vi "SHA-1.vi"(1 "Data":u8[](array[numeric])) -> (0 "message-digest":u8[](array[numeric]))   [LabVIEW 2016, in "websocket upgrade handler.lvclass"]
uses:
  websocket upgrade handler.lvclass
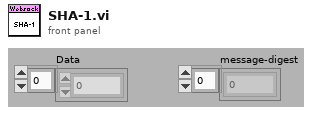
[diagram p1: front panel]
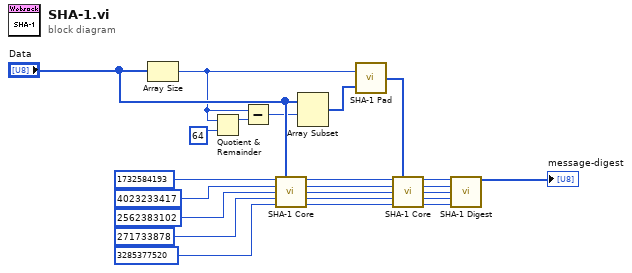
[diagram p0: block diagram]
diagram:
  n1 = Array Size(array="Data") -> (size(s)=w1:i32)
  n2 = Quotient & Remainder(x=w1, y=64) -> (x-y*floor(x/y)=w12:i32)  [unwired: 1 out]
  n3 = Subtract(x=w1, y=w12) -> (x-y=w18:i32)
  n4 = call "SHA-1 Core.vi"("s1"=u32 1732584193, "Input Bytes"="Data", "s2"=u32 4023233417, "s3"=u32 2562383102, "s4"=u32 271733878, "s5"=u32 3285377520 ("s4")) -> ("s1 out"=w13:u32, "s2 out"=w14:u32, "s3 out"=w15:u32, "s4 out"=w16:u32, "s5 out"=w17:u32)  [unwired: 5 in]
  n5 = Array Subset(array="Data", index=w18) -> (w19:u8[])  [unwired: 1 in]
  n6 = call "SHA-1 Pad.vi"("Last Part"=w19, "Message Length (bytes)"=w1) -> ("Padding"=w20:u8[])
  n7 = call "SHA-1 Core.vi"("s1"=w13, "Input Bytes"=w20, "s2"=w14, "s3"=w15, "s4"=w16, "s5"=w17) -> ("s1 out"=w6:u32, "s2 out"=w5:u32, "s3 out"=w4:u32, "s4 out"=w3:u32, "s5 out"=w2:u32)  [unwired: 5 in]
  n8 = call "SHA-1 Digest.vi"("s1"=w6, "s2"=w5, "s3"=w4, "s4"=w3, "s5"=w2) -> ("message-digest"=→"message-digest":u8[])  [unwired: 10 in]
